vi "GEOM_GetAvailableReadModes.vi"(8 "error in (no error)":errorcluster) -> (0 "error out":errorcluster, 2 "info":string)   [LabVIEW 2016]
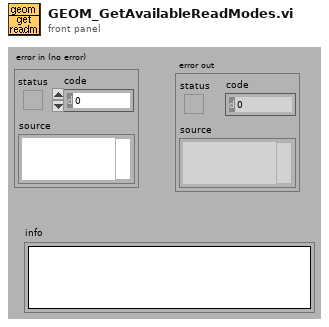
[diagram p1: front panel]
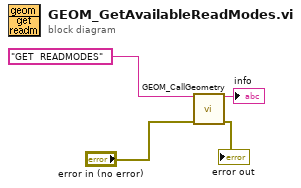
[diagram p0: block diagram]
diagram:
  n1 = call "GEOM_CallGeometry.vi"("Command"="GET  READMODES" ("string (\"\")"), "error in (no error)"="error in (no error)") -> ("ImmedReplyString"=→"info":string, "error out"=→"error out":errorcluster)  [unwired: 12 out]
